vi "QSM-PC (String)__slk_QSM-PC (String).vi"(9 "user event out":refnum<user-event>, 11 "event registration refnum":refnum<event-registration>) -> ()   [LabVIEW 2015, in "QSM-PC (String).lvlib"]
uses:
  Library/QSM-PC (String).lvlib
panel:
  in  "Stop Button":bool
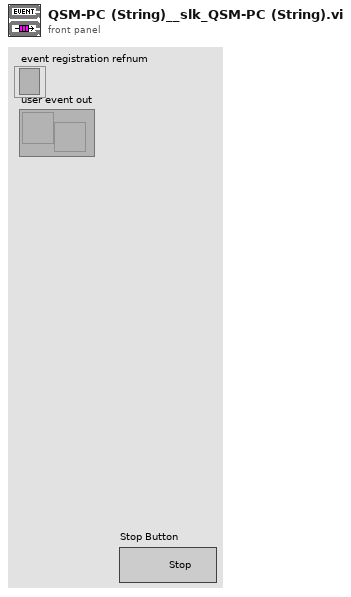
[diagram p1: front panel]
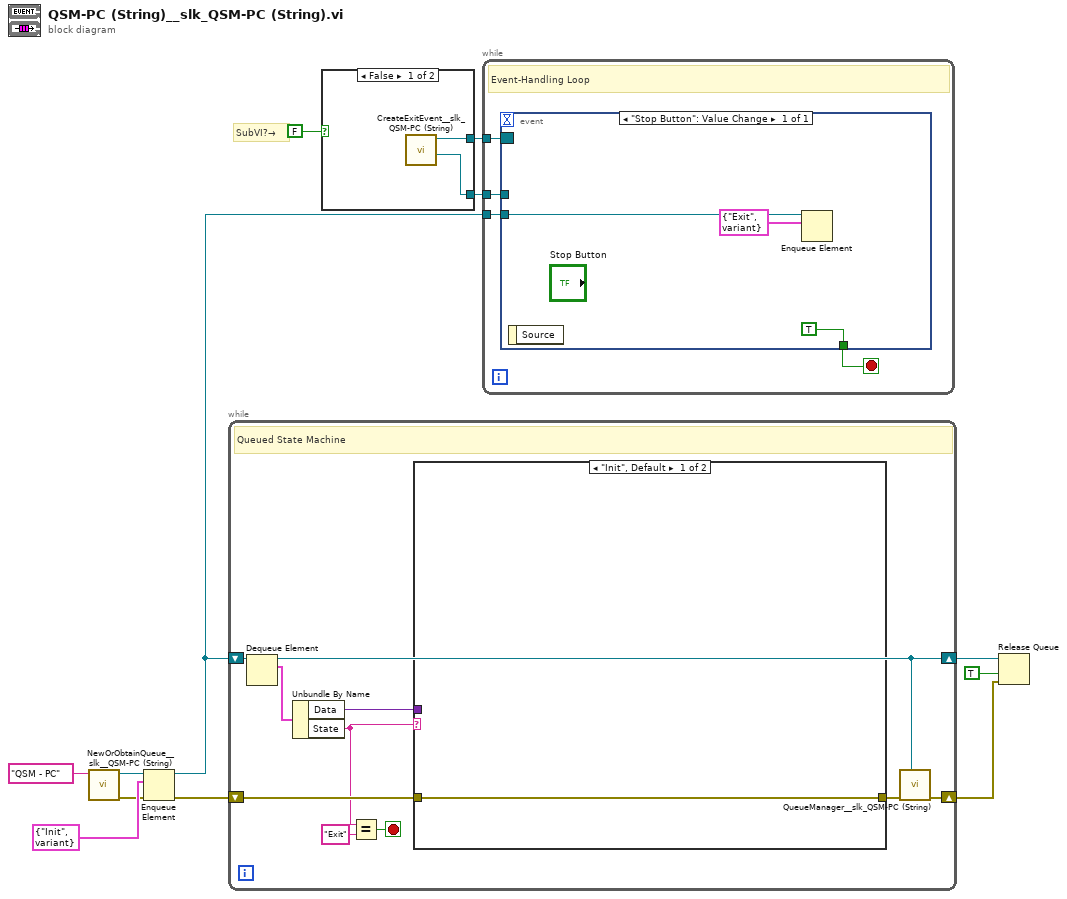
[diagram p0: block diagram]
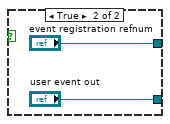
[diagram p2: hidden frame]
diagram:
  # "SubVI?→"
  n1 = call "NewOrObtainQueue__slk__QSM-PC (String).vi"("queue name in"="QSM - PC" ("name (unnamed)")) -> ("error out"=w2:errorcluster, "queue out"=w8:refnum<queue>)  [unwired: 2 in, 7 out]
  n2 = Enqueue Element(queue=w8, element=cluster{"State":string, "Data":variant} {"State"="Init", "Data"=variant} ("Element"), error in (no error)=w2) -> (queue out=w4:refnum<queue>, error out=w7:errorcluster)  [unwired: 2 out]
  n3 = while {
    shift-right: [w15] -> w1
    shift-left: w7 -> [w19]
    shift-right: [w16] -> w6
    shift-left: w4 -> [w22]
    stop <- w17 stop-if-true
    # "Queued State Machine"
    n4 = Dequeue Element(queue=w22) -> (queue out=w16:refnum<queue>, element=w21:cluster{"State":string, "Data":variant})  [unwired: 1 in, 3 out]
    n5 = Unbundle By Name(w21) -> ("Data"=w20:variant, "State"=w18:string)
    n6 = Equal?(x=w18, y="Exit") -> (x = y?=w17:bool)
    n7 = case shown="\"Init\", Default" w18 {
      tunnel: w20 -> [_ _]
      tunnel: w19 -> [w23 _]
      tunnel: [w23 _] -> w14
      frame "Init", Default {
      }
      frame "IDLE" {
      }
    }
    n8 = call "QueueManager__slk_QSM-PC (String).vi"("queue in"=w16, "error in (no error)"=w14) -> ("error out"=w15:errorcluster)  [unwired: 2 in, 7 out]
  }
  n9 = case shown="False" FALSE {
    tunnel: [w25 "event registration refnum"] -> w12
    tunnel: [w24 "user event out"] -> w11
    frame False {
      n10 = call "CreateExitEvent__slk_QSM-PC (String).vi"() -> ("user event out"=w24:refnum<user-event>, "event registration refnum out"=w25:refnum<event-registration>)  [unwired: 10 out]
    }
    frame True {
    }
  }
  n11 = while {
    tunnel: w12 -> [w31]
    tunnel: w11 -> [w30]
    tunnel: w4 -> [w29]
    stop <- w28 stop-if-true
    # "Event-Handling Loop"
    n12 = event shown="[0] \"Stop Button\": Value Change" {
      selector: w31 -> [_]
      dyn-events: _ -> [_]
      timeout: _ -> [_]
      tunnel: w30 -> [_]
      tunnel: w29 -> [w34]
      tunnel: [TRUE] -> w28
      event "Stop Button": Value Change {
        n13 = event-data() -> ()  [unwired: 2 out]
        n14 = Enqueue Element(queue=w34, element=cluster{"State":string, "Data":variant} {"State"="Exit", "Data"=variant} ("Element")) -> ()  [unwired: 1 in, 4 out]
      }
    }
  }
  n15 = Release Queue(queue=w6, force destroy? (F)=TRUE, error in (no error)=w1) -> ()  [unwired: 3 out]
